vi "UI - Initiate Connection.vi"(8 "error in (no error)":errorcluster caption="错误输入（无错误）", 10 "Controller Address":string caption="控制器地址", 11 "Message Queue":refnum<queue> caption="消息队列") -> (0 "error out":errorcluster caption="错误输出", 1 "Connected?":bool caption="已连接？")   [LabVIEW 2013]
uses:
  Message Queue/Message Cluster.ctl
  controls/Control State.ctl
  controls/Variable References.ctl
  Globals/Global - Configuration Options.vi
  Globals/Global - UI Stream and Variable Connections.vi
  Message Queue/Message Queue.lvlib
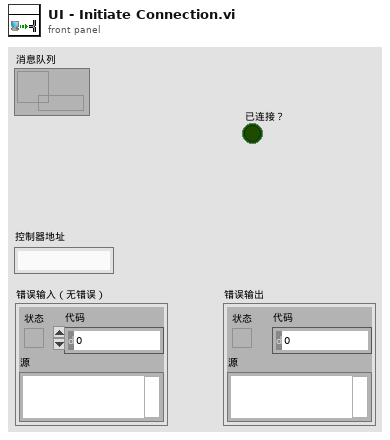
[diagram p1: front panel]
types:
  T1 = typedef "Control State.ctl" = enum16{"Safe State", "Manual", "Control (PID)"}
  T2 = typedef "Message Queue.lvlib/Message Cluster.ctl" = cluster{"Message":string, "Message Data":variant}
  T3 = typedef "Variable References.ctl" = cluster{"CPU Usage":refnum<k21>, "Contiguous Memory":refnum<k21>, "Control Mode":refnum<k21>, "Control Loop Period":refnum<k21>, "Input Values":refnum<k21>, "Output Values":refnum<k21>}
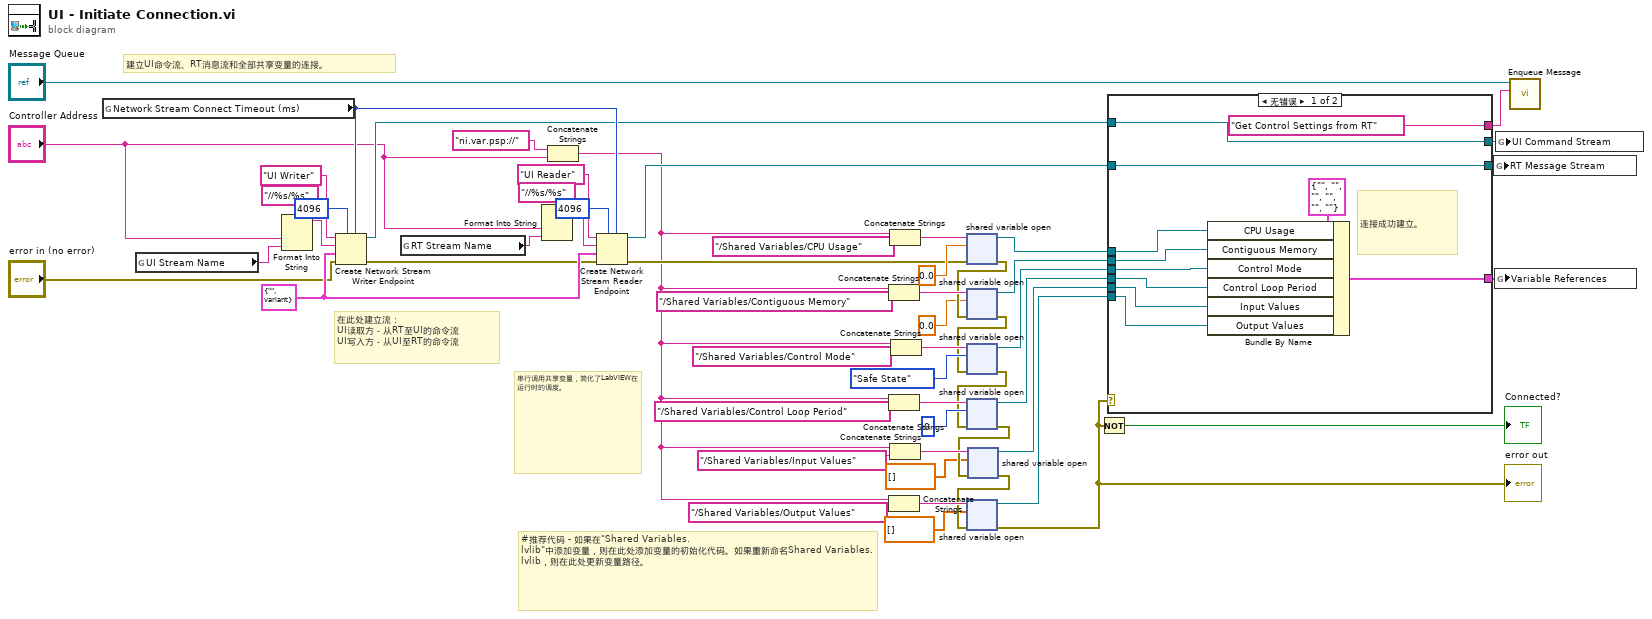
[diagram p0: block diagram]
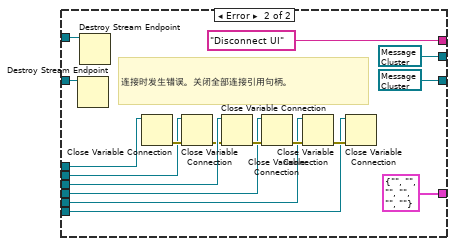
[diagram p2: hidden frame]
diagram:
  w47 = T2 {"Message"="", "Message Data"=variant} ("Message Cluster")
  # "建立UI命令流、RT消息流和全部共享变量的连接。"
  # "#推荐代码 - 如果在\"Shared Variables.lvlib\"中添加变量，则在此处添加变量的初始化代码。如果重新命名Shared Variables.lvlib，则在此处更新变量路径。"
  # "在此处建立流：\nUI读取方－从RT至UI的命令流\nUI写入方－从UI至RT的命令流"
  # "串行调用共享变量，简化了LabVIEW在运行时的调度。"
  n1 = global read "Global - Configuration Options.vi" "Network Stream Connect Timeout (ms)"() -> (w46:i32)
  n2 = global read "Global - Configuration Options.vi" "UI Stream Name"() -> (w54:string)
  n3 = Format Into String(format string="//%s/%s", "Controller Address", w54) -> (resulting string=w53:string)  [unwired: 2 in, 1 out]
  n4 = Create Network Stream Writer Endpoint(5:w46, 7:4096 ("writer buffer size"), 8:"error in (no error)", 9:w47, 10:w53, 11:"UI Writer" ("writer name")) -> (0:w19:errorcluster, 3:w27:refnum<k21>)  [unwired: 1 in]
  n5 = global read "Global - Configuration Options.vi" "RT Stream Name"() -> (w51:string)
  n6 = Format Into String(format string="//%s/%s", "Controller Address", w51) -> (resulting string=w50:string)  [unwired: 2 in, 1 out]
  n7 = Concatenate Strings("ni.var.psp://", "Controller Address") -> (w11:string)
  n8 = Create Network Stream Reader Endpoint(5:w46, 7:4096 ("reader buffer size"), 8:w19, 9:w47, 10:w50, 11:"UI Reader" ("reader name")) -> (0:w18:errorcluster, 3:w26:refnum<k21>)  [unwired: 1 in]
  n9 = Concatenate Strings(w11, "/Shared Variables/Contiguous Memory") -> (w40:string)
  n10 = Concatenate Strings(w11, "/Shared Variables/Control Loop Period") -> (w36:string)
  n11 = Concatenate Strings(w11, "/Shared Variables/Output Values") -> (w12:string)
  n12 = Concatenate Strings(w11, "/Shared Variables/CPU Usage") -> (w43:string)
  n13 = Concatenate Strings(w11, "/Shared Variables/Input Values") -> (w15:string)
  n14 = Concatenate Strings(w11, "/Shared Variables/Control Mode") -> (w39:string)
  n15 = shared-variable-open(w43, w18, 0.0) -> (w31:refnum<k21>, w33:errorcluster)  [unwired: 1 in]
  n16 = shared-variable-open(w40, w33, 0.0) -> (w30:refnum<k21>, w17:errorcluster)  [unwired: 1 in]
  n17 = shared-variable-open(w39, w17, Control_State."Safe State" ("FPGA State")) -> (w29:refnum<k21>, w32:errorcluster)  [unwired: 1 in]
  n18 = shared-variable-open(w36, w32, u32 0) -> (w28:refnum<k21>, w10:errorcluster)  [unwired: 1 in]
  n19 = shared-variable-open(w15, w10, dbl[] []) -> (w5:refnum<k21>, w9:errorcluster)  [unwired: 1 in]
  n20 = shared-variable-open(w12, w9, dbl[] []) -> (w4:refnum<k21>, w8:errorcluster)  [unwired: 1 in]
  "error out" <- w8
  n21 = Not(x=w8) -> (.not. x?=→"Connected?":bool)
  n22 = case shown="无错误" w8 {
    tunnel: w31 -> [w66 w80]
    tunnel: w30 -> [w65 w77]
    tunnel: w29 -> [w64 w78]
    tunnel: w28 -> [w63 w79]
    tunnel: w27 -> [w59 w83]
    tunnel: w26 -> [w61 w84]
    tunnel: [w62 T3 {"CPU Usage"="", "Contiguous Memory"="", "Control Mode"="", "Control Loop Period"="", "Input Values"="", "Output Values"=""} ("Variable References")] -> w25
    tunnel: [w61 refnum<k21> refnum] -> w24
    tunnel: [w59 refnum<k21> refnum] -> w23
    tunnel: ["Get Control Settings from RT" "Disconnect UI"] -> w21
    tunnel: w5 -> [w58 w69]
    tunnel: w4 -> [w57 w68]
    frame No Error {
      # "连接成功建立。"
      n23 = Bundle By Name(cluster=T3 {"CPU Usage"="", "Contiguous Memory"="", "Control Mode"="", "Control Loop Period"="", "Input Values"="", "Output Values"=""} ("Variable References"), "CPU Usage"=w66, "Contiguous Memory"=w65, "Control Mode"=w64, "Control Loop Period"=w63, "Input Values"=w58, "Output Values"=w57) -> (w62:T3)
    }
    frame Error {
      # "连接时发生错误。关闭全部连接引用句柄。"
      n24 = Destroy Stream Endpoint(11:w84) -> ()  [unwired: 1 in, 1 out]
      n25 = Destroy Stream Endpoint(11:w83) -> ()  [unwired: 1 in, 1 out]
      n26 = Close Variable Connection(11:w80) -> (0:w81:errorcluster)  [unwired: 1 in]
      n27 = Close Variable Connection(8:w81, 11:w77) -> (0:w72:errorcluster)
      n28 = Close Variable Connection(8:w72, 11:w78) -> (0:w82:errorcluster)
      n29 = Close Variable Connection(8:w82, 11:w79) -> (0:w71:errorcluster)
      n30 = Close Variable Connection(8:w71, 11:w69) -> (0:w70:errorcluster)
      n31 = Close Variable Connection(8:w70, 11:w68) -> ()  [unwired: 1 out]
    }
  }
  n32 = global write "Global - UI Stream and Variable Connections.vi" "RT Message Stream"(w24) -> ()
  n33 = global write "Global - UI Stream and Variable Connections.vi" "Variable References"(w25) -> ()
  n34 = global write "Global - UI Stream and Variable Connections.vi" "UI Command Stream"(w23) -> ()
  n35 = call "Enqueue Message.vi"("Message"=w21, "Message Queue"="Message Queue") -> ()  [unwired: 8 in, 2 out]
